vi "ScaleRead.vi"(8 "error in (no error)":errorcluster, 11 "VISA Refnum in":refnum<visa-resource-name>) -> (0 "error out":errorcluster, 2 "Numeric":dbl, 3 "VISA Refnum out":refnum<visa-resource-name>)   [LabVIEW 2023]
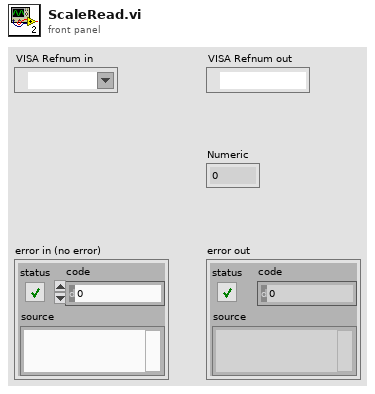
[diagram p1: front panel]
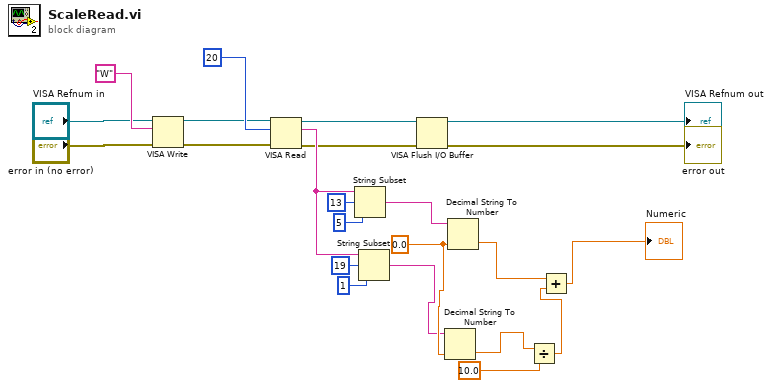
[diagram p0: block diagram]
diagram:
  w23 = 0.0 ("default (0 I32)")
  n1 = VISA Write(VISA resource name="VISA Refnum in", write buffer="W", error in (no error)="error in (no error)") -> (VISA resource name out=w4:refnum<visa-resource-name>, error out=w2:errorcluster)  [unwired: 1 out]
  n2 = VISA Read(VISA resource name=w4, byte count=u32 20, error in (no error)=w2) -> (VISA resource name out=w8:refnum<visa-resource-name>, read buffer=w16:string, error out=w10:errorcluster)  [unwired: 1 out]
  n3 = String Subset(string=w16, offset (0)=13, length (rest)=5 ("length (rest)")) -> (substring=w12:string)
  n4 = String Subset(string=w16, offset (0)=19, length (rest)=1 ("length (rest)")) -> (substring=w17:string)
  n5 = VISA Flush I/O Buffer(VISA resource name=w8, error in (no error)=w10) -> (VISA resource name out=→"VISA Refnum out":refnum<visa-resource-name>, error out=→"error out":errorcluster)  [unwired: 1 in]
  n6 = Decimal String To Number(string=w17, default (0L)=w23) -> (number=w19:dbl)  [unwired: 1 in, 1 out]
  n7 = Decimal String To Number(string=w12, default (0L)=w23) -> (number=w18:dbl)  [unwired: 1 in, 1 out]
  n8 = Divide(x=w19, y=sgl 10.0) -> (x/y=w21:dbl)
  n9 = Add(x=w18, y=w21) -> (x+y=→"Numeric":dbl)
